vi "Practica 13 - Programa Principal LDK.vi"() -> ()   [LabVIEW 2023]
panel:
  out "I10":dbl
  out "I7":dbl
  out "I6":dbl
  out "I4":dbl
  out "I2":dbl
  out "I1":dbl
  out "I7":bool
  out "I2":bool
  out "I6":bool
  out "I4":bool
  out "I10":bool
  out "I1":bool
  out "R10":dbl
  out "R8 Y R9":dbl
  out "R7":dbl
  out "R5 Y R6":dbl
  out "R3 Y R4":dbl
  out "R1 Y  R2":dbl
  out "R11 Y R12":dbl
  in  "R11":dbl
  in  "R6":dbl
  in  "R1":dbl
  in  "R12":dbl
  in  "R10":dbl
  in  "R3":dbl
  in  "R5":dbl
  in  "R4":dbl
  in  "VOLTAGE":dbl
  in  "R2":dbl
  in  "R9":dbl
  in  "R8":dbl
  in  "R7":dbl
  # "LEYES DE KIRCHHOFF"
  # "VOLTAJE EN RESISTENCIAS"
  # "Corriente en mallas"
  # "MALLA 3"
  # "MALLA 2"
  # "MALLA 1"
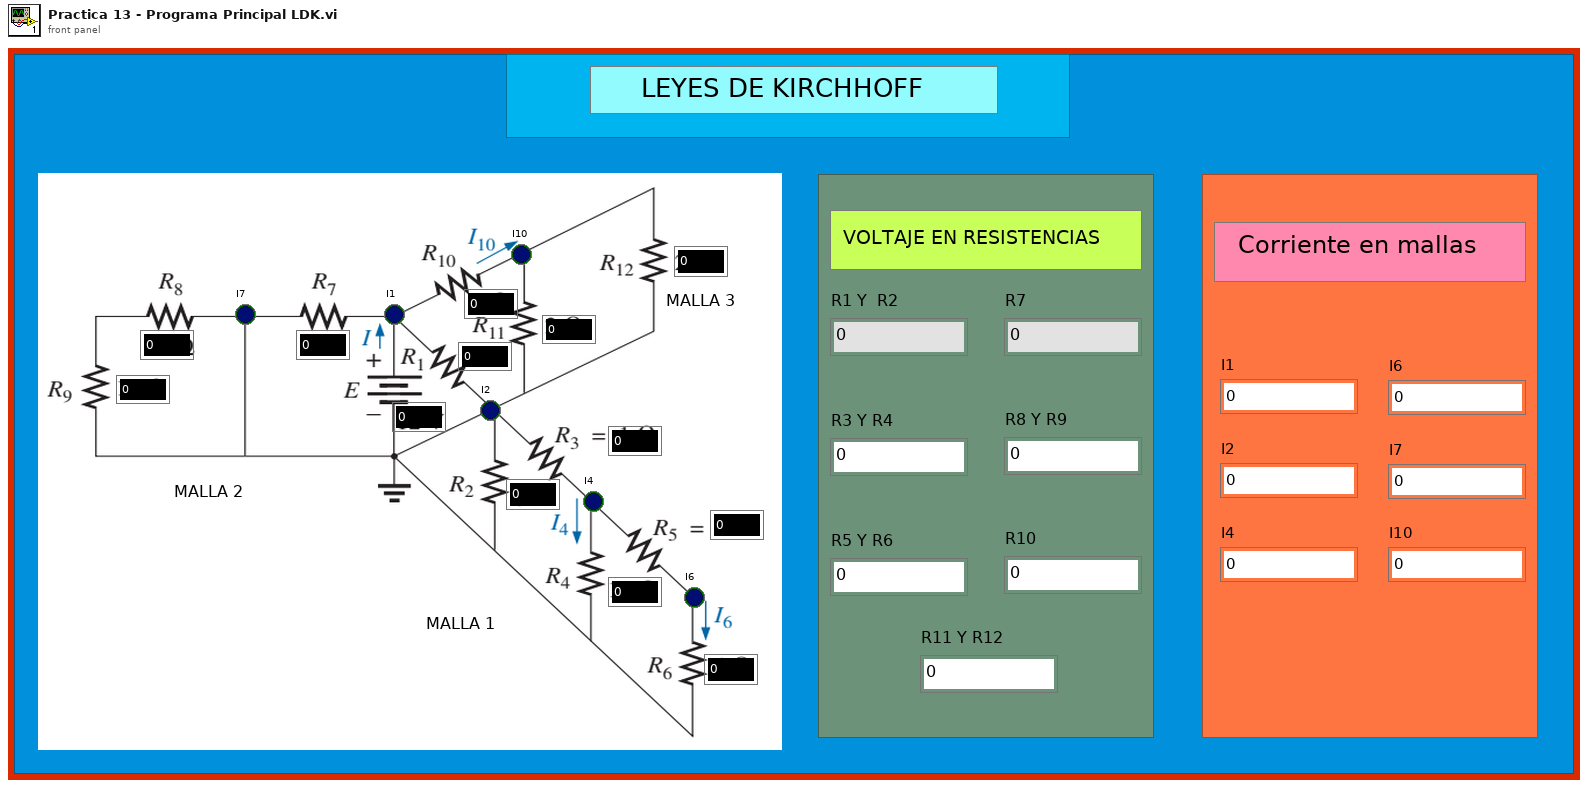
[diagram p1: front panel]
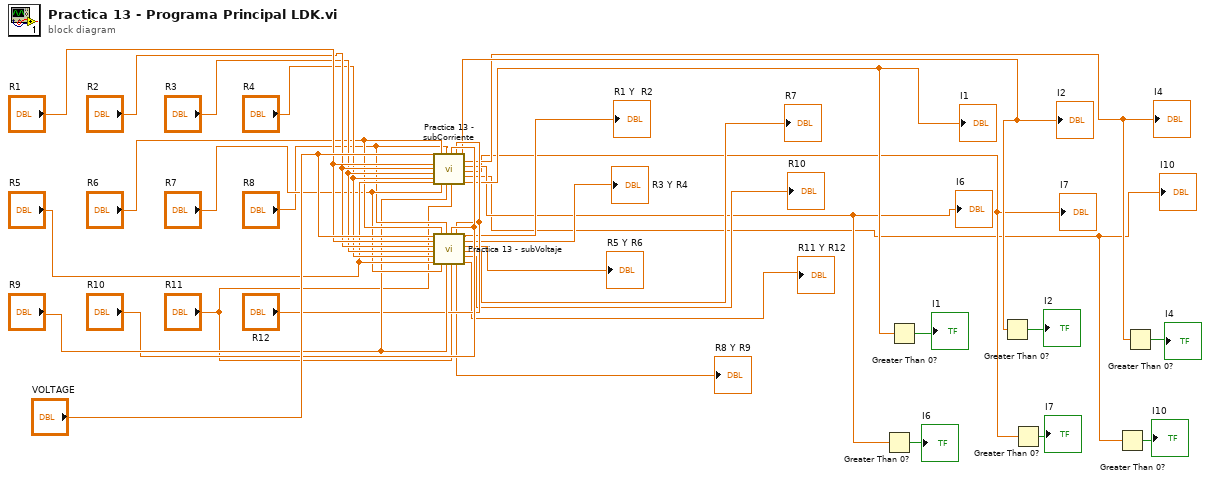
[diagram p0: block diagram]
diagram:
  n1 = call "Practica 13 - subCorriente.vi"("VOLTAGE"="VOLTAGE", "R1"="R1", "R2"="R2", "R3"="R3", "R4"="R4", "R5"="R5", "R6"="R6", "R7"="R7", "R8"="R8", "R9"="R9", "R10"="R10", "R11"="R11", "R12"="R12") -> ("MALLA 1A"=w9:dbl, "MALLA 1B"=w7:dbl, "MALLA 1C"=w5:dbl, "MALLA 2"=w3:dbl, "MALLA 3"=w1:dbl, "CORRIENTE TOTAL"=w11:dbl)  [unwired: 1 in]
  "I1" <- w11
  "I2" <- w9
  "I4" <- w7
  "I6" <- w5
  "I7" <- w3
  "I10" <- w1
  n2 = call "Practica 13 - subVoltaje.vi"("VOLTAGE"="VOLTAGE", "R1"="R1", "R2"="R2", "R3"="R3", "R4"="R4", "R5"="R5", "R6"="R6", "R7"="R7", "R8"="R8", "R9"="R9", "R10"="R10", "R11"="R11", "R12"="R12") -> ("VOLTAJE R8 R9"=→"R8 Y R9":dbl, "VOLTAJE R1 R2"=→"R1 Y  R2":dbl, "VOLTAJE R3 R4"=→"R3 Y R4":dbl, "VOLTAJE R5 R6"=→"R5 Y R6":dbl, "VOLTAJE R7"=→"R7":dbl, "VOLTAJE R10"=→"R10":dbl, "VOLTAJE R11 R12"=→"R11 Y R12":dbl)
  n3 = Greater Than 0?(x=w5) -> (x > 0?=→"I6":bool)
  n4 = Greater Than 0?(x=w11) -> (x > 0?=→"I1":bool)
  n5 = Greater Than 0?(x=w9) -> (x > 0?=→"I2":bool)
  n6 = Greater Than 0?(x=w3) -> (x > 0?=→"I7":bool)
  n7 = Greater Than 0?(x=w1) -> (x > 0?=→"I10":bool)
  n8 = Greater Than 0?(x=w7) -> (x > 0?=→"I4":bool)
